vi "CLD 15 Text String Parsing Front Panel.vi"(8 "Fehler (Eingang)":T2) -> (0 "Fehler (Ausgang)":T2)   [LabVIEW 2014]
doc: "CLD-Übung 15"
uses:
  CLD 15 CSV file data structure.ctl
  Zustaende.ctl
  <vilib>/Utility/file.llb/Write To Spreadsheet File (string).vi
  <vilib>/Utility/file.llb/Read From Spreadsheet File (string).vi
panel:
  in  "Stopp":bool
  out "Daten":string[][](array[string])
  out "In Datei gespeicherte Daten":string[][](array[string])
  out "Verarbeitete Daten":T1[](array[typedef])
  # "Verarbeitete Daten"
  # "Eingangsdaten"
  # "Ausgangsdaten"
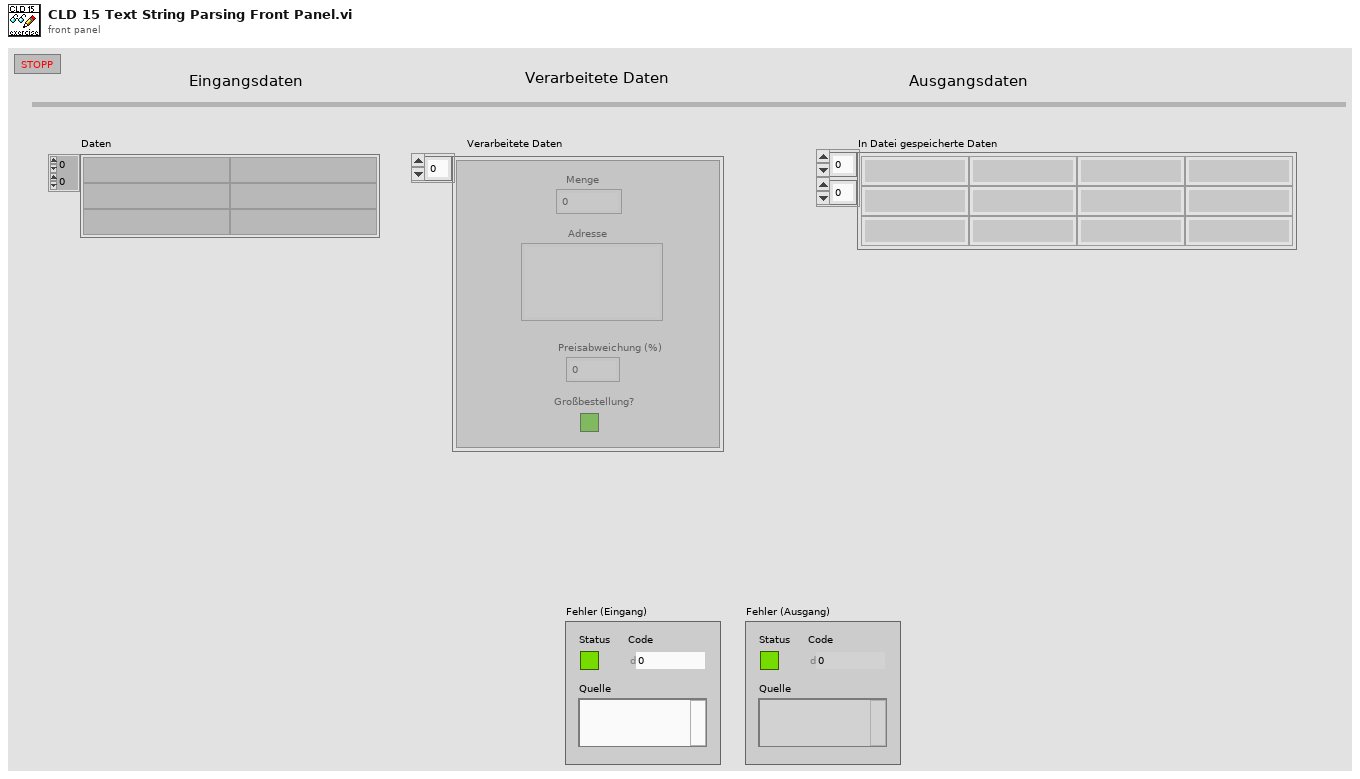
[diagram p1: front panel]
types:
  T1 = typedef "CLD 15 CSV file data structure.ctl" = cluster{"Menge":i32, "Adresse":string, "Preisabweichung (%)":dbl, "Großbestellung?":bool}
  T2 = cluster{"Status":bool, "Code":i32, "Quelle":string}
  T3 = typedef "Zustaende.ctl" = enum16{"Initialisieren", "Beenden", "Ergebnis speichern", "Ergebnis anzeigen", "Datei anzeigen", "Datei parsen", "Datei einlesen", "Datei öffnen", "Idle"}
  T4 = enum16{"open", "replace", "create", "open or create", "replace or create", "replace or create with confirmation"}
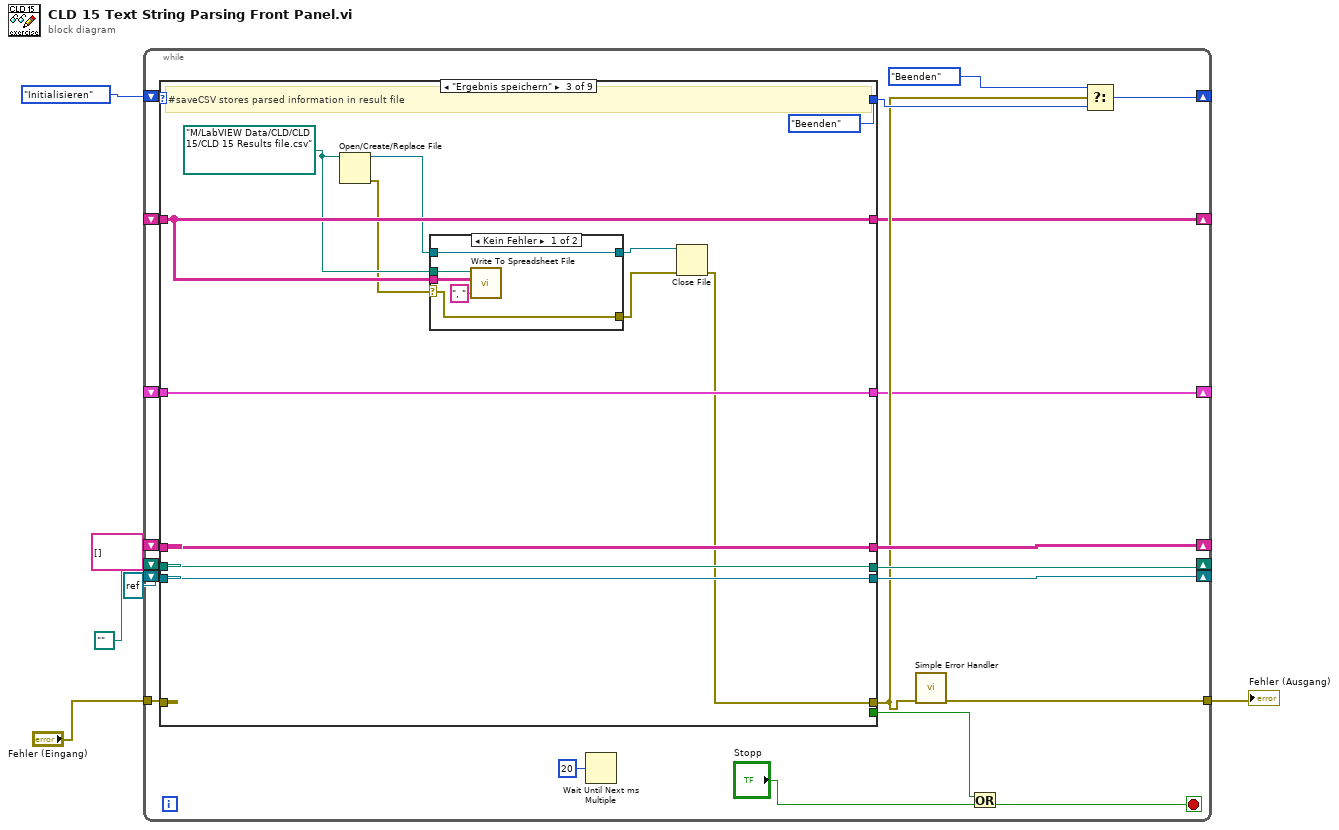
[diagram p0: block diagram]
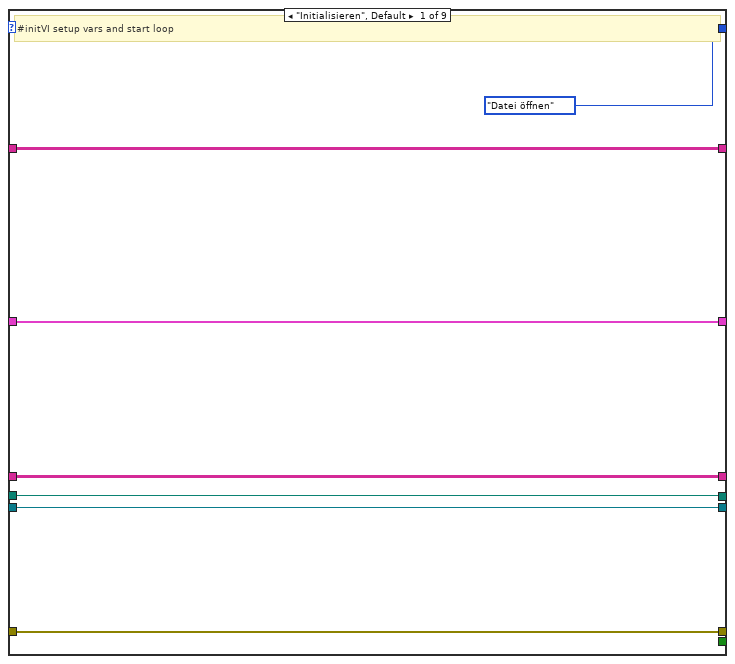
[diagram p2: hidden frame]
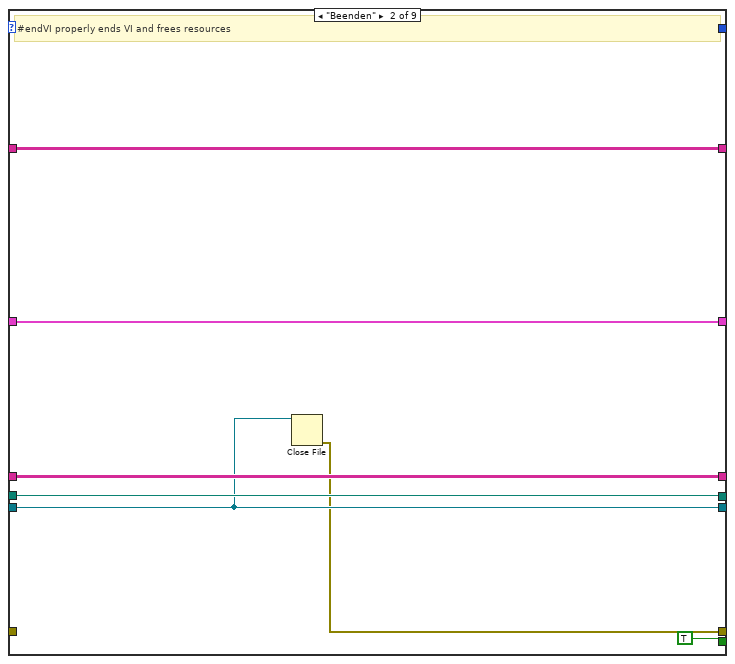
[diagram p3: hidden frame]
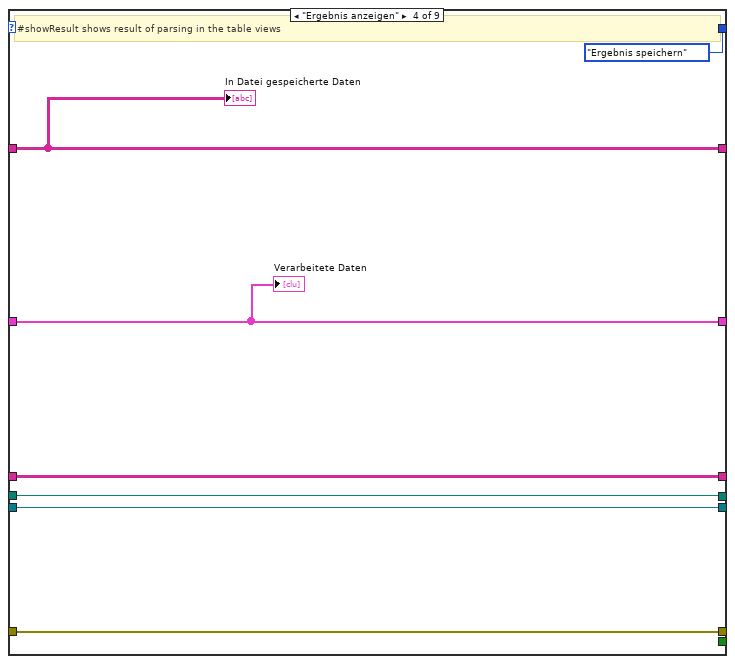
[diagram p5: hidden frame]
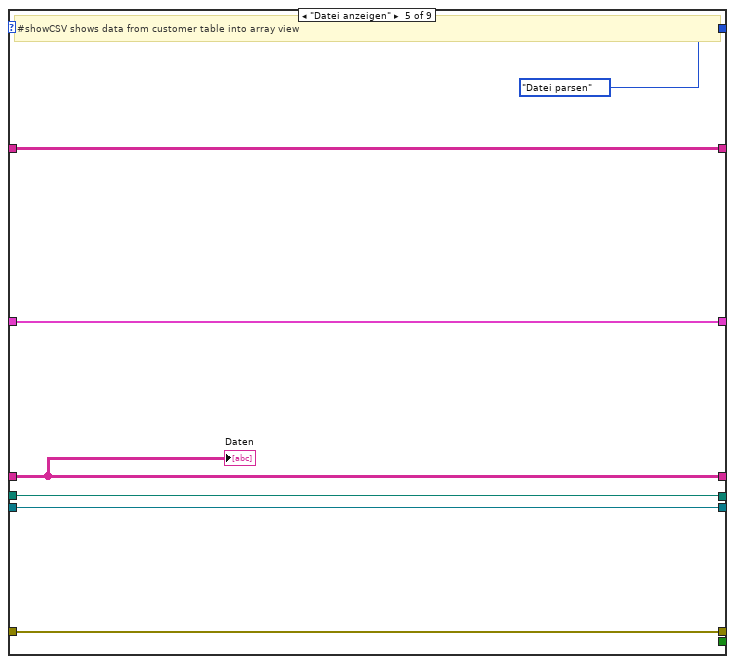
[diagram p6: hidden frame]
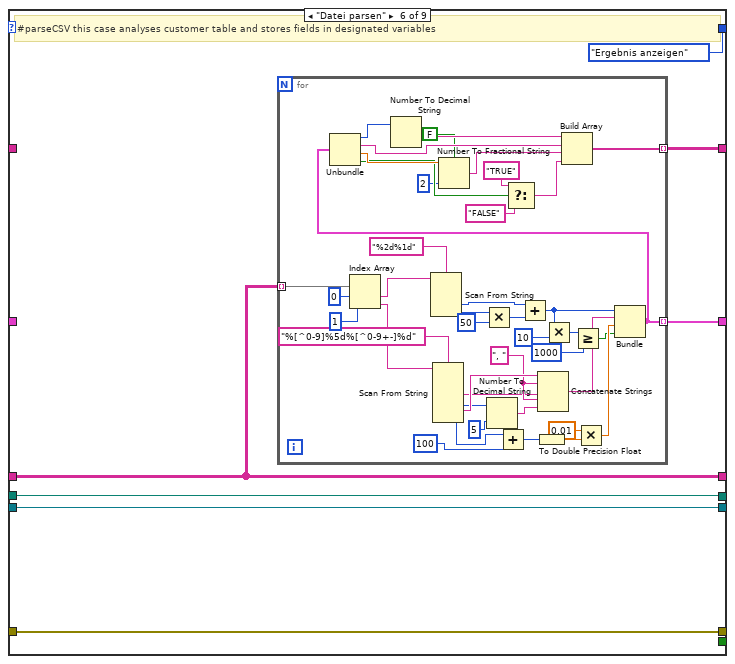
[diagram p7: hidden frame]
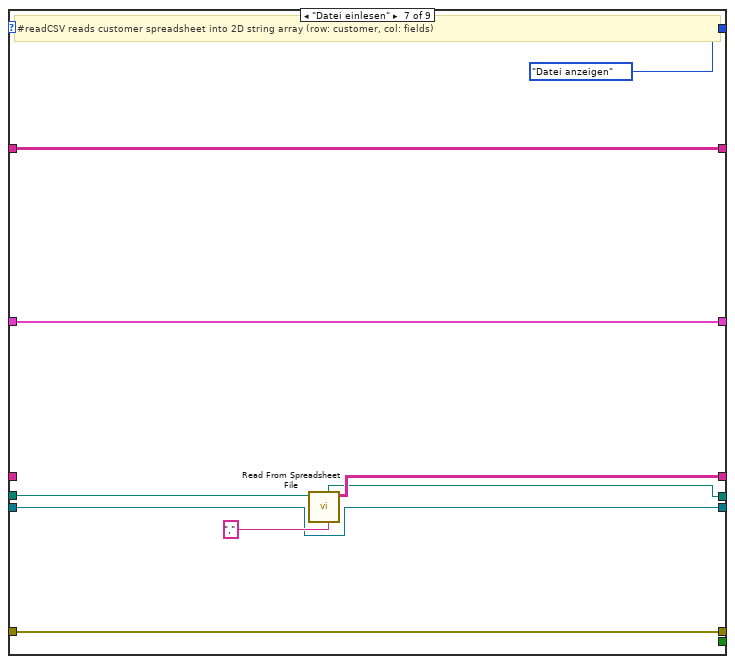
[diagram p8: hidden frame]
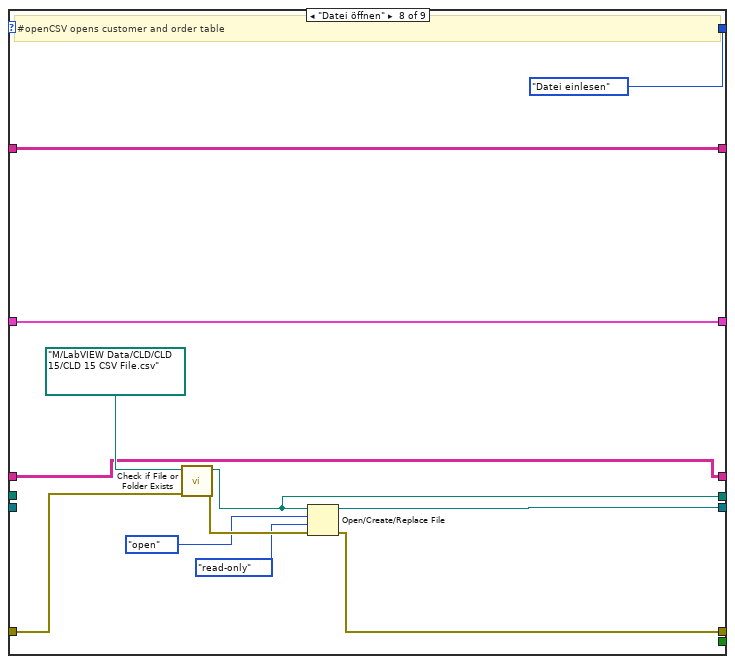
[diagram p9: hidden frame]
diagram:
  n1 = while {
    tunnel: "Fehler (Eingang)" -> [w26]
    shift-right: [w25] -> _
    shift-left: refnum<file> refnum ("refnum out") -> [w24]
    shift-right: [w23] -> _
    shift-left: path "" ("dup path") -> [w22]
    shift-right: [w21] -> _
    shift-left: string[][] [] ("all rows") -> [w20]
    shift-right: [w15] -> _
    shift-left: Zustaende."Initialisieren" -> [w27]
    tunnel: [w19] -> w4
    shift-right: [w11] -> _
    shift-left: _ -> [w10]
    shift-right: [w9] -> _
    shift-left: _ -> [w8]
    stop <- w14 stop-if-true
    n2 = case shown="\"Ergebnis speichern\"" w27 {
      selector: w27 -> [_ _ _ _ _ _ _ _ w147]
      tunnel: w26 -> [w34 _ _ w67 w74 w81 w132 w140 w151]
      tunnel: [w34 w38 w43 w67 w74 w81 w132 w141 w151] -> w12
      tunnel: [w31 w39 w52 w64 w71 w79 w128 w144 w150] -> w25
      tunnel: w24 -> [w31 w39 w52 w64 w71 w79 w128 _ w150]
      tunnel: [w32 w40 w51 w65 w72 w80 w126 w139 w149] -> w23
      tunnel: w22 -> [w32 w40 w51 w65 w72 w80 w131 _ w149]
      tunnel: [w33 w41 w53 w66 w73 w78 w130 w138 w148] -> w21
      tunnel: w20 -> [w33 w41 w53 w66 w73 w78 _ w138 w148]
      tunnel: [Zustaende."Datei öffnen" _ Zustaende."Beenden" Zustaende."Ergebnis speichern" Zustaende."Datei parsen" Zustaende."Ergebnis anzeigen" Zustaende."Datei anzeigen" Zustaende."Datei einlesen" w147] -> w17
      tunnel: [_ TRUE _ _ _ _ _ _ _] -> w13
      tunnel: [w29 w36 w50 w63 w69 w76 w125 w134 w146] -> w11
      tunnel: w10 -> [w29 w36 w50 w63 w69 _ w125 w134 w146]
      tunnel: [w28 w35 w49 w61 w68 w75 w124 w133 w145] -> w9
      tunnel: w8 -> [w28 w35 w49 w61 w68 _ w124 w133 w145]
      frame "Initialisieren", Default {
        # "#initVI setup vars and start loop"
      }
      frame "Beenden" {
        # "#endVI properly ends VI and frees resources"
        n3 = Close File(refnum=w39) -> (error out=w38:errorcluster)  [unwired: 1 in, 1 out]
      }
      frame "Ergebnis speichern" {
        w48 = path "M:/LabVIEW Data/CLD/CLD 15/CLD 15 Results file.csv" ("file path (dialog if empty)")
        # "#saveCSV stores parsed information in result file"
        n4 = Open/Create/Replace File(file path (use dialog)=w48) -> (refnum out=w46:refnum<file>, error out=w47:errorcluster)  [unwired: 5 in, 1 out]
        n5 = case shown="Kein Fehler" w47 {
          selector: w47 -> [w55 w60]
          tunnel: w49 -> [w58 _]
          tunnel: w48 -> [w56 _]
          tunnel: [w55 w60] -> w44
          tunnel: w46 -> [w54 w59]
          tunnel: [w54 w59] -> w45
          frame No Error {
            n6 = call-poly <vilib>:"Write To Spreadsheet File.vi"("delimiter (\\t)"=", " ("delimiter (\\t)"), "2D data"=w58, "file path (dialog if empty)"=w56) -> ()  [unwired: 5 in, 1 out]
          }
          frame Error {
          }
        }
        n7 = Close File(refnum=w45, error in=w44) -> (error out=w43:errorcluster)  [unwired: 1 out]
      }
      frame "Ergebnis anzeigen" {
        # "#showResult shows result of parsing in the table views"
        "Verarbeitete Daten" <- w63
        "In Datei gespeicherte Daten" <- w61
      }
      frame "Datei anzeigen" {
        # "#showCSV shows data from customer table into array view"
        "Daten" <- w73
      }
      frame "Datei parsen" {
        # "#parseCSV this case analyses customer table and stores fields in designated variables"
        n8 = for {
          tunnel: w78 -> [w123] mode=indexing
          tunnel: [w88] -> w76 mode=indexing
          tunnel: [w84] -> w75 mode=indexing
          w111 = ", " ("String")
          n9 = Index Array(array=w123, index #1=0 ("Index"), index #2=1 ("Index")) -> (element #1=w120:string, element #2=w118:string)
          n10 = Scan From String(format string="%2d%1d" ("Format-String"), input string=w120) -> (output 1=w114:i32, output 2=w116:i32)  [unwired: 4 in, 3 out]
          n11 = Scan From String(format string="%[^0-9]%5d%[^0-9+-]%d" ("Format-String"), input string=w118) -> (output 1=w110:string, output 2=w108:i32, output 3=w112:string, output 4=w105:i32)  [unwired: 6 in, 3 out]
          n12 = Multiply ("Multiplizieren")(x=w116, y=50) -> (x*y=w113:i32)
          n13 = Number To Decimal String(number=w108, width (-)=i16 5 ("Breite (-)")) -> (decimal integer string=w109:string)
          n14 = Add(x=w105, y=100) -> (x+y=w103:i32)
          n15 = Add(x=w114, y=w113) -> (x+y=w99:i32)
          n16 = To Double Precision Float(number=w103) -> (double precision float=w101:dbl)
          n17 = Concatenate Strings(w112, w111, w110, w111, w109) -> (w106:string)
          n18 = Multiply ("Multiplizieren")(x=w99, y=10) -> (x*y=w97:i32)
          n19 = Greater Or Equal?(x=w97, y=1000) -> (x >= y?=w95:bool)
          n20 = Multiply(x=0.01, y=w101) -> (x*y=w100:dbl)
          n21 = Bundle(w99, w106, w100, w95) -> (w88:cluster{i32, string, dbl, bool})  [unwired: 1 in]
          n22 = Unbundle(w88) -> (w89:i32, w92:string, w90:dbl, w85:bool)
          n23 = Number To Decimal String(number=w89) -> (decimal integer string=w91:string)  [unwired: 1 in]
          n24 = Number To Fractional String(use system decimal point (T)=FALSE ("Systemdezimalzeichen verwenden (T)"), number=w90, precision (6)=i16 2 ("Genauigkeit (6)")) -> (F-format string=w93:string)  [unwired: 1 in]
          n25 = Select(t="TRUE", s=w85, f="FALSE") -> (s? t:f=w86:string)
          n26 = Build Array(w91, w92, w93, w86) -> (w84:string[])
        }
      }
      frame "Datei einlesen" {
        # "#readCSV reads customer spreadsheet into 2D string array (row: customer, col: fields)"
        n27 = call-poly <vilib>:"Read From Spreadsheet File.vi"("delimiter (\\t)"="," ("delimiter (\\t)"), "file path (dialog if empty)"=w131) -> ("all rows"=w130:string[][], "new file path (Not A Path if cancelled)"=w126:path)  [unwired: 5 in, 3 out]
      }
      frame "Datei öffnen" {
        # "#openCSV opens customer and order table"
        n28 = call <vilib>:"Check if File or Folder Exists.vi"("error in (no error)"=w140, "path"=path "M:/LabVIEW Data/CLD/CLD 15/CLD 15 CSV File.csv" ("Dateipfad (Dialog verwenden)")) -> ("error out"=w142:errorcluster, "dup path"=w139:path)  [unwired: 7 in, 1 out]
        n29 = Open/Create/Replace File(file path (use dialog)=w139, error in=w142, operation (0:open)=T4."open" ("Operation (0:Öffnen)"), access (0:read/write)=enum16{"read/write", "read-only", "write-only"}."read-only" ("Zugriff (0:Lesen/Schreiben)")) -> (refnum out=w144:refnum<file>, error out=w141:errorcluster)  [unwired: 2 in, 1 out]
      }
      frame "Idle" {
        # "#idle do noting"
      }
    }
    n30 = Wait Until Next ms Multiple(millisecond multiple=u32 20 ("ms")) -> ()  [unwired: 1 out]
    n31 = call <vilib>:"Simple Error Handler.vi"("error in (no error)"=w12) -> ("error out"=w19:errorcluster)  [unwired: 4 in, 4 out]
    n32 = Or(x=w13, y="Stopp") -> (x .or. y?=w14:bool)
    n33 = Select(t=Zustaende."Beenden" ("f"), s=w12, f=w17) -> (s? t:f=w15:T3)
  }
  "Fehler (Ausgang)" <- w4
